vi "Delete Oneof Template Files.vi"(8 "error in (no error)":errorcluster, 11 "Library in":refnum<vi>) -> (0 "error out":errorcluster, 3 "Library out":refnum<vi>)   [LabVIEW 2019, in "gRPC Template Creation Utility.lvlib"]
uses:
  gRPC Template Creation Utility.lvlib
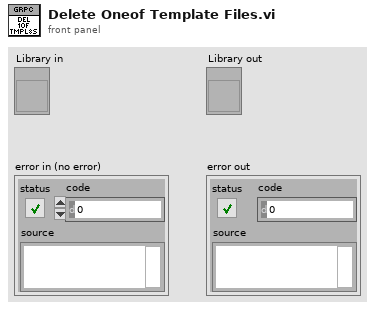
[diagram p1: front panel]
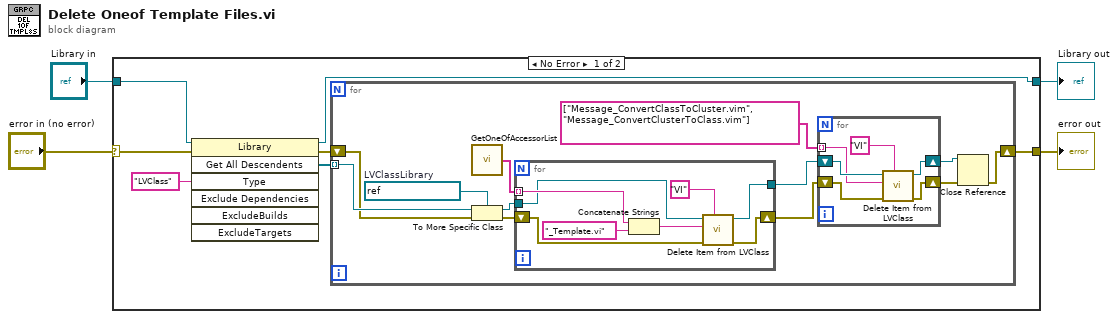
[diagram p0: block diagram]
diagram:
  n1 = case shown="No Error" "error in (no error)" {
    selector: "error in (no error)" -> [w6 w39]
    tunnel: "Library in" -> [w8 w38]
    tunnel: [w7 w38] -> w3
    tunnel: [w5 w39] -> w1
    frame No Error {
      n2 = invoke class="Library" method="Get All Descendents"(reference=w8, error in=w6, "Type"="LVClass") -> (reference out=w7:refnum<vi>, error out=w11:errorcluster, "All Descendents"=w10:refnum<vi>[])  [unwired: 4 in, 4 out]
      n3 = for {
        tunnel: w10 -> [w22] mode=indexing
        shift-right: [w17] -> w5
        shift-left: w11 -> [w19]
        w21 = refnum<vi> refnum  # LVClassLibrary
        n4 = call "GetOneOfAccessorList.vi"() -> ("Array"=w23:string[])
        n5 = To More Specific Class(target class=w21, reference=w22, error in=w19) -> (specific class reference=w20:refnum<vi>, error out=w18:errorcluster)
        n6 = for {
          tunnel: w23 -> [w37] mode=indexing
          tunnel: w20 -> [w35]
          shift-right: [w31] -> w14
          shift-left: w18 -> [w32]
          tunnel: [w30] -> w16
          n7 = Concatenate Strings(w37, "_Template.vi" ("string")) -> (w34:string)
          n8 = call "Delete Item from LVClass.vi"("Item Type"="VI", "error in (no error)"=w32, "Item name"=w34, "LVClassLibrary in"=w35) -> ("error out"=w31:errorcluster, "LVClassLibrary out"=w30:refnum<vi>)  [unwired: 5 in, 1 out]
        }
        n9 = for {
          shift-right: [w28] -> w15
          shift-left: w16 -> [w29]
          shift-right: [w26] -> w13
          shift-left: w14 -> [w27]
          tunnel: string[] ["Message_ConvertClassToCluster.vim", "Message_ConvertClusterToClass.vim"] -> [w25] mode=indexing
          n10 = call "Delete Item from LVClass.vi"("Item Type"="VI", "error in (no error)"=w27, "Item name"=w25, "LVClassLibrary in"=w29) -> ("error out"=w26:errorcluster, "LVClassLibrary out"=w28:refnum<vi>)  [unwired: 5 in, 1 out]
        }
        n11 = Close Reference(reference=w15, error in (no error)=w13) -> (error out=w17:errorcluster)
      }
    }
    frame Error {
    }
  }
  "Library out" <- w3
  "error out" <- w1
